vi "XNET Subframe Property Node.vi"   [LabVIEW 2018]
doc: "Property node used to read/write properties for an XNET Subframe I/O name."
uses:
  <resource>/objmgr/xnet.rc
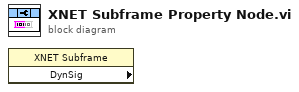
[diagram p0: block diagram]
diagram:
  n1 = property class="XNET Subframe" props=["DynSig"]() -> ()  [unwired: 2 in, 3 out]
